vi "configuration UI.vi"() -> ()   [LabVIEW 2013, in "control module editor.lvclass"]
uses:
  control module editor.lvclass
  <vilib>/NI/Configuration Framework/Node/NodeRef.ctl
  <vilib>/NI/Configuration Framework/Node/NISE_CEF_Node.lvclass
  <vilib>/NI/AMC/Message Queue.ctl
  <vilib>/NI/AMC/Message.ctl
  <vilib>/NI/Tools/Keyed Array/KeyedArray.ctl
  <vilib>/NI/Configuration Framework/Node/UserEventRef.ctl
  <vilib>/NI/Configuration Framework/Controls/EventCluster.ctl
  configuration/error classification setting.ctl
  <vilib>/NI/Tag Bus Module Framework/runtime/error classification.ctl
  <vilib>/NI/Configuration Framework/Node/RefreshUIEvent.ctl
  <vilib>/NI/Configuration Framework/Node/CacheState.ctl
  <vilib>/NI/Configuration Framework/Node/StopEvent.ctl
  <vilib>/NI/Configuration Framework/Node/NodeChangeEvent.ctl
  configuration/control module configuration.lvclass
  <vilib>/NI/Configuration Framework/serializable configuration/NISE_CEF_serializable configuration.lvclass/NISE_CEF_serializable configuration.ctl
  <vilib>/NI/Configuration Framework/serializable configuration/NISE_CEF_serializable configuration.lvclass
  configuration/control module configuration.lvclass/control module configuration.ctl
  <vilib>/NI/Tag Bus Module Framework/module configuration/TBM module configuration.lvclass
  <vilib>/NI/Tag Bus Module Framework/channel/TBM channel.lvclass
  <vilib>/NI/Tag Bus/tag/tag descriptor.lvclass/tag descriptor.ctl
  <vilib>/NI/Tag Bus Module Framework/channel/channel classification.ctl
  <vilib>/NI/Configuration Framework/serializable configuration/Read UID.vi
  configuration/Read error classifications.vi
  configuration/Write error classifications.vi
  read fixed channel configuration.vi
  Configuration Editor/Classes/Module editor node/Read Module Configuration.vi
  <vilib>/NI/Module Execution Interface/Engine Configuration/engine configuration.lvclass
  <vilib>/NI/Tag Bus/tag/tag descriptor.lvclass
  <vilib>/NI/Configuration Framework/NISE_CEF_TreeControl.lvlib
  Configuration Editor/Classes/Engine Parent/Engine Parent Editor Node.lvclass
  Configuration Editor/Classes/Module editor node/module editor node.lvclass
  <vilib>/NI/Tools/Keyed Array/Tools_KeyedArray.lvlib
  <vilib>/NI/AMC/AMC.lvlib
  <vilib>/NI/Tag Bus Module Framework/runtime/TBM module execution interface.lvclass
panel:
  in  "node change":T1
  in  "stop event":T2
  in  "cache state":T3
  in  "refresh UI":T4
  in  "Tab Control":T5(tab)
  in  "mapwriters":bool
  out "Channel List":string[][](table)
  in  "mapall":bool
  in  "kvp":i32(listbox)
  in  "error classifications":T6[](array[typedef])
  in  "user event":T8
  in  "main queue":T9
  in  "node ref":T10
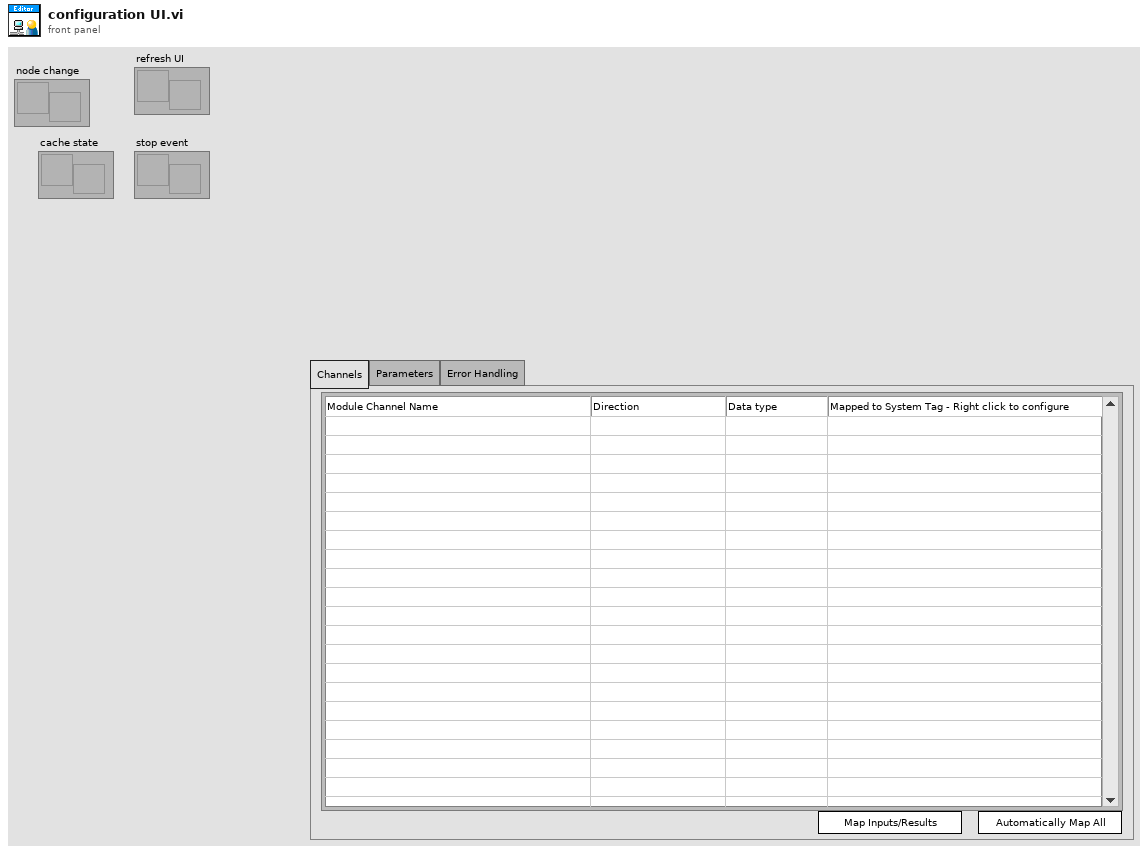
[diagram p1: front panel]
types:
  T1 = typedef "NISE_CEF_Node.lvclass/NodeChangeEvent.ctl" = refnum<user-event>
  T2 = typedef "NISE_CEF_Node.lvclass/StopEvent.ctl" = refnum<user-event>
  T3 = typedef "NISE_CEF_Node.lvclass/CacheState.ctl" = refnum<user-event>
  T4 = typedef "NISE_CEF_Node.lvclass/RefreshUIEvent.ctl" = refnum<user-event>
  T5 = enum32{"Channels", "Parameters", "Error Handling"}
  T6 = typedef "control module configuration.lvclass/error classification setting.ctl" = cluster{"code":i32, "error classification":T7}
  T7 = typedef "TBM module execution interface.lvclass/error classification.ctl" = enum16{"unknown", "none", "trivial", "recoverable", "critical"}
  T8 = typedef "NISE_CEF_Node.lvclass/UserEventRef.ctl" = refnum<user-event>
  T9 = typedef "AMC.lvlib/Message Queue.ctl" = refnum<queue>
  T10 = typedef "NISE_CEF_Node.lvclass/NodeRef.ctl" = refnum<data-value>
  T11 = typedef "control module configuration.lvclass/error classification.ctl" = cluster{"code":i32, "error classification":T7}
  T12 = typedef "NISE_CEF_TreeControl.lvlib/EventCluster.ctl" = cluster{"command":string, "data":string}
  T13 = typedef "LVPoint32TypeDef.ctl" = cluster{"Horizontal":i32, "Vertical":i32}
  T14 = typedef "LVRowAndColumnTypeDef.ctl" = cluster{"Row":i32, "Column":i32}
  T15 = typedef "TBM channel.lvclass/channel classification.ctl" = enum16{"input data", "output data", "processing parameter", "processing result"}
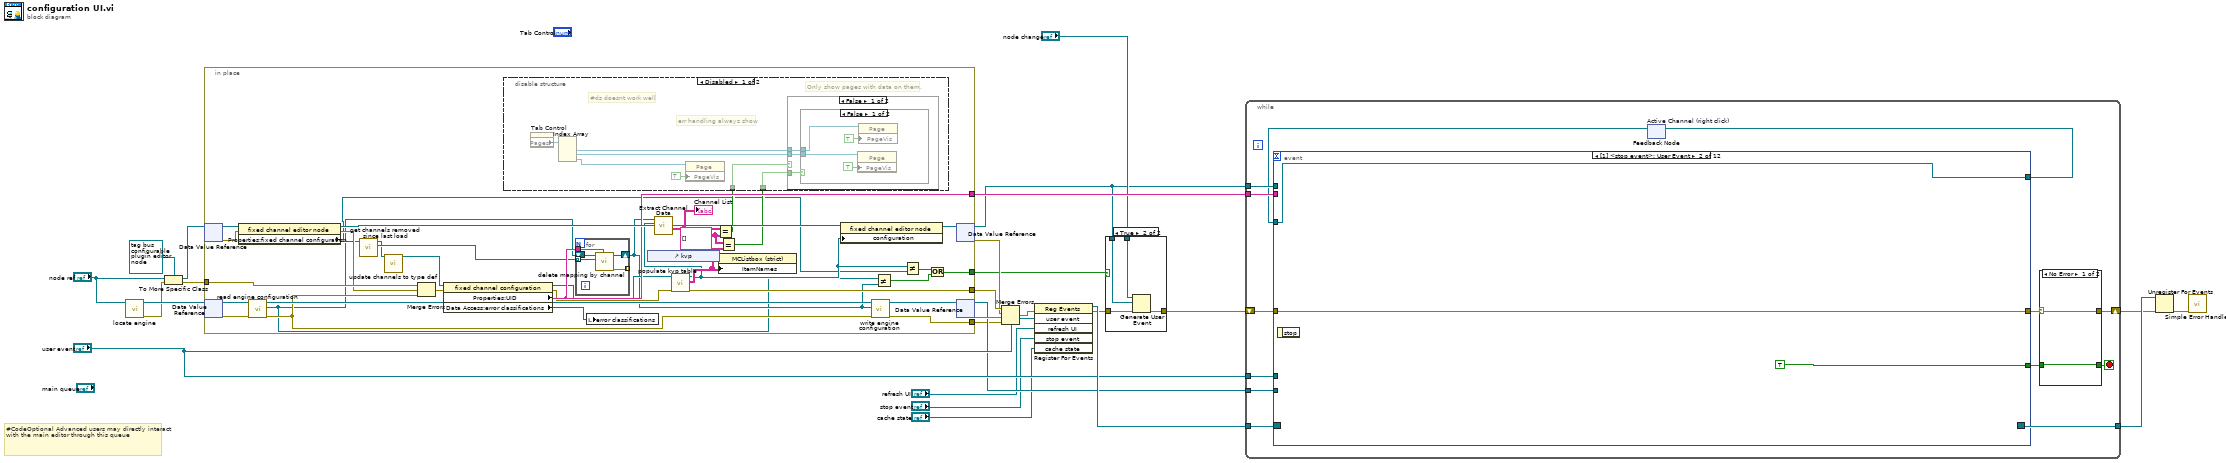
[diagram p0: block diagram]
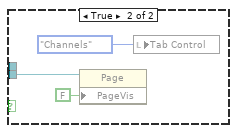
[diagram p3: hidden frame]
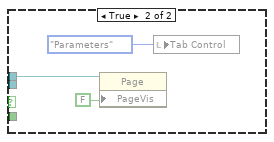
[diagram p4: hidden frame]
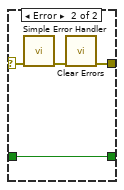
[diagram p6: hidden frame]
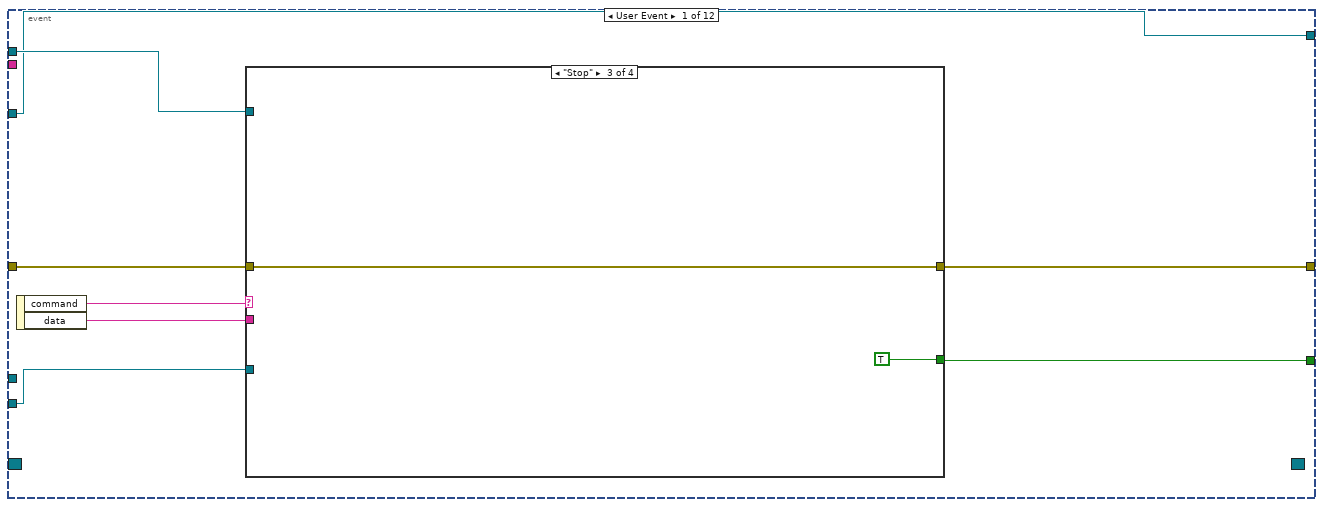
[diagram p7: hidden frame]
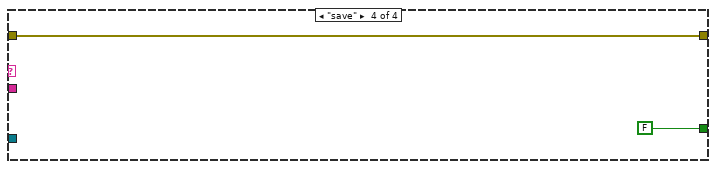
[diagram p10: hidden frame]
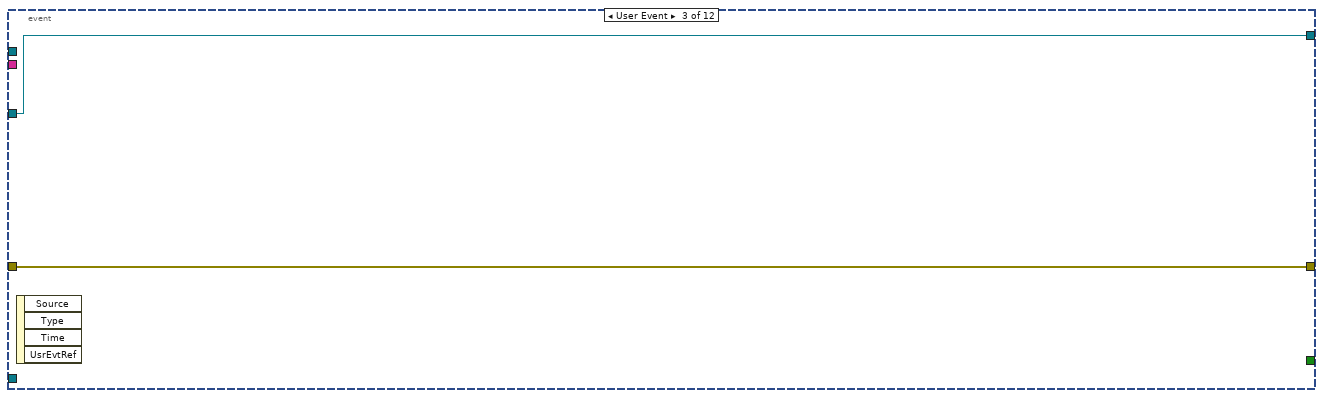
[diagram p11: hidden frame]
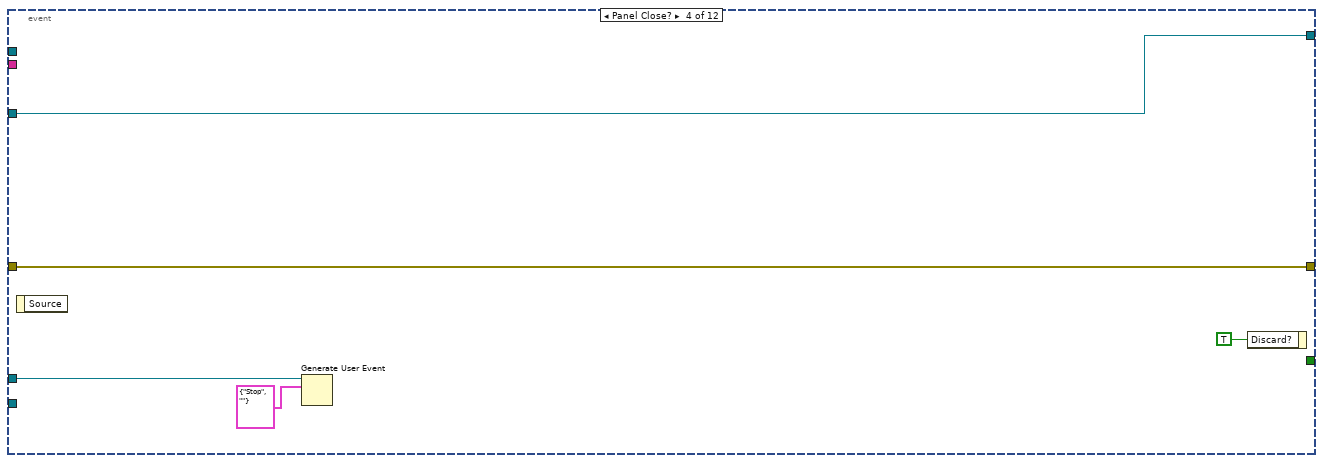
[diagram p12: hidden frame]
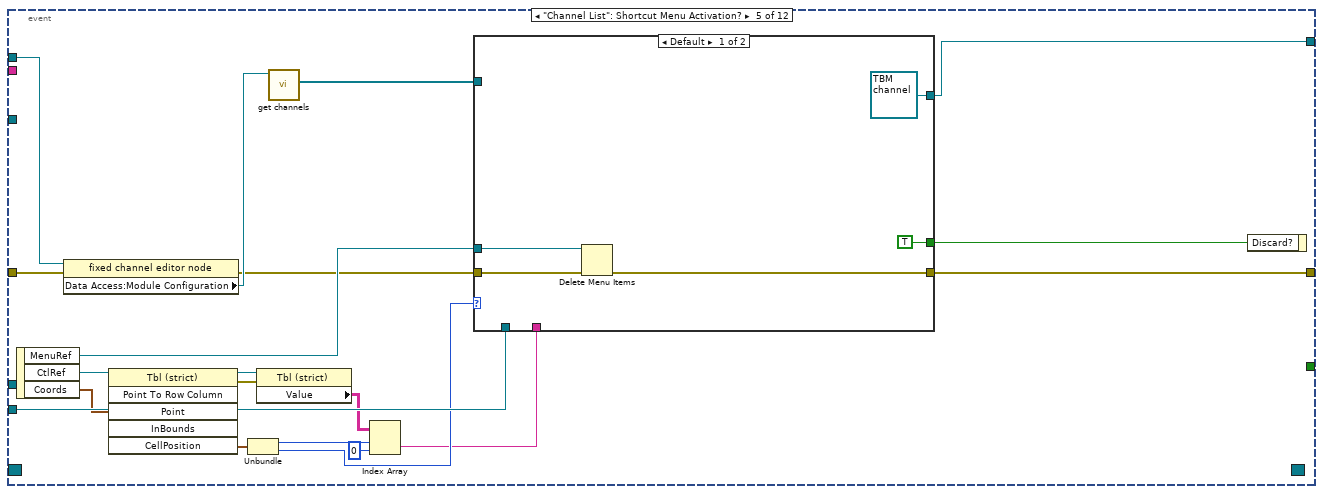
[diagram p13: hidden frame]
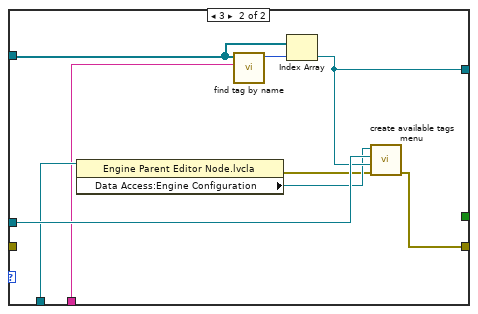
[diagram p14: hidden frame]
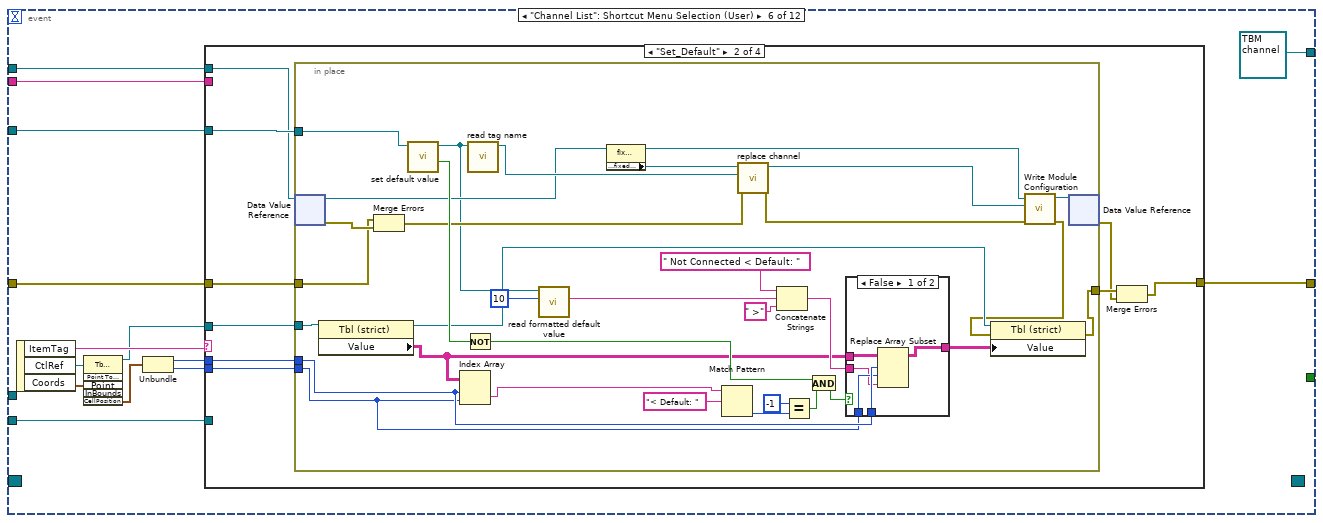
[diagram p15: hidden frame]
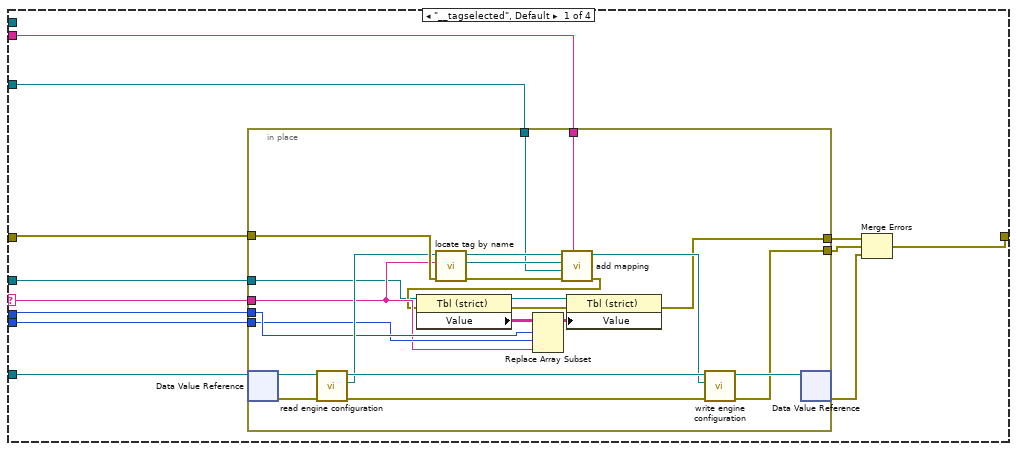
[diagram p16: hidden frame]
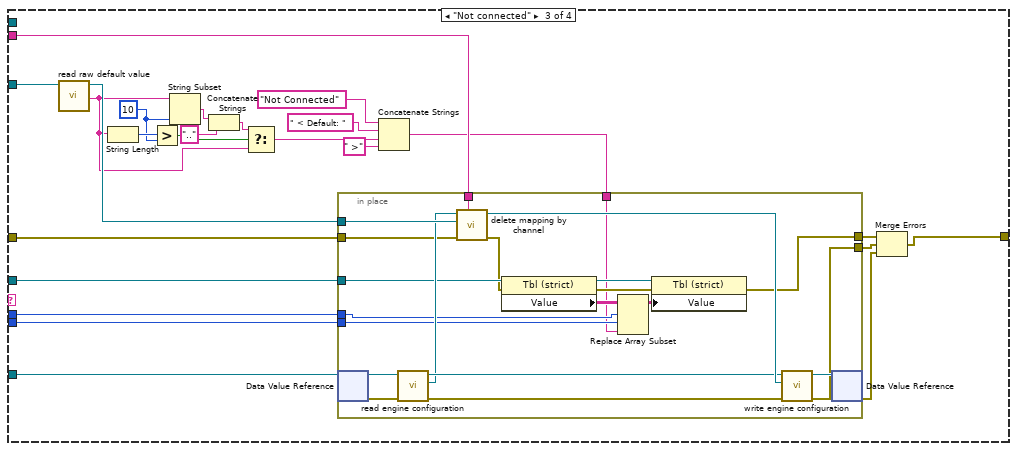
[diagram p18: hidden frame]
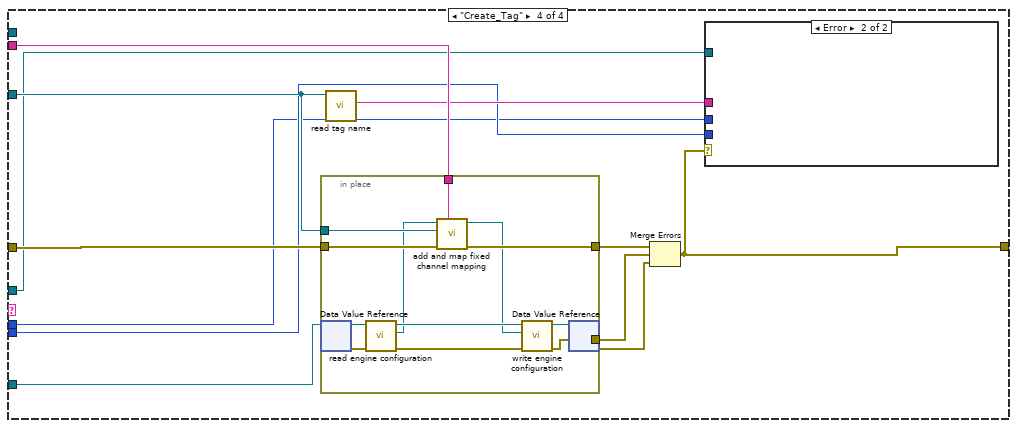
[diagram p19: hidden frame]
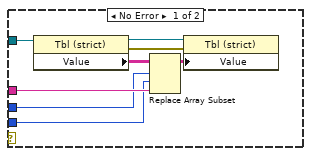
[diagram p20: hidden frame]
diagram:
  # "#CodeOptional Advanced users may directly interact with the main editor through this queue"
  n1 = call "locate engine.vi"("component"="node ref") -> ("error out"=w9:errorcluster, "engine"=w11:refnum<data-value>)  [unwired: 9 in]
  n2 = To More Specific Class(target class=refnum<data-value> refnum ("data value reference"), reference="node ref", error in=w9) -> (specific class reference=w19:refnum<data-value>, error out=w18:errorcluster)
  n3 = in-place {
    in-place-border: w18 -> [w60]
    in-place-border: [w54] -> w17
    in-place-border: [w51] -> w13
    in-place-border: [w35] -> w3
    in-place-border: [w27] -> w2
    w44 = string[][] [] ("y")
    n4 = in-place-dvr #1(w19) -> (w57:refnum<class "control module editor.lvclass">, w52:errorcluster)
    n5 = in-place-dvr #2(w11) -> (w59:refnum<class "Engine Parent Editor Node.lvclass">, w55:errorcluster)
    n6 = property class="fixed channel editor node"(reference=w57, error in=w52) -> (reference out=w53:refnum<class "control module editor.lvclass">, error out=w48:errorcluster, "Properties:fixed channel configuration"=w32:refnum<class "control module configuration.lvclass">)
    n7 = call "read engine configuration.vi"("error in"=w55, "Engine Parent Editor Node in"=w59) -> ("error out"=w36:errorcluster, "engine configuration"=w30:refnum<class "engine configuration.lvclass">, "Engine Parent Editor Node out"=w58:refnum<class "Engine Parent Editor Node.lvclass">)  [unwired: 7 in]
    n8 = call "get channels removed since last load.vi"("fixed channel configuration in"=w32) -> ("removed"=w50:refnum<class "TBM channel.lvclass">[], "fixed channel configuration out"=w40:refnum<class "control module configuration.lvclass">)  [unwired: 9 in]
    n9 = call-dynamic "update channels to type def.vi"("fixed channel configuration in"=w40) -> ("fixed channel configuration out"=w39:refnum<class "control module configuration.lvclass">)  [unwired: 10 in]
    n10 = Merge Errors(w60, w48, w36) -> (w56:errorcluster)
    n11 = property class="fixed channel configuration"(reference=w39, error in=w56) -> (reference out=w34:refnum<class "control module configuration.lvclass">, error out=w49:errorcluster, "Properties:UID"=w51:string, "Data Access:error classifications"=w38:T11[])
    n12 = for {
      tunnel: w51 -> [w85]
      tunnel: w50 -> [w84] mode=indexing
      shift-right: [w83] -> w31
      shift-left: w30 -> [w82]
      tunnel: [w81] -> _ mode=indexing
      n13 = call <vilib>:"delete mapping by channel.vi"("owner ID"=w85, "channel"=w84, "engine configuration in"=w82) -> ("error out"=w81:errorcluster, "engine configuration out"=w83:refnum<class "engine configuration.lvclass">)  [unwired: 7 in]
    }
    n14 = local write "error classifications"(w38) -> ()
    n15 = control-ref of="kvp"() -> (w47:refnum<vi>)
    n16 = call "populate kvp table.vi"("error in"=w49, "fixed channel configuration in"=w34) -> ("error out"=w54:errorcluster, "kvp's"=w43:string[][], "fixed channel configuration out"=w33:refnum<class "control module configuration.lvclass">)  [unwired: 7 in]
    n17 = call "Extract Channel Data.vi"("module configuration in"=w33, "Engine Configuration"=w31) -> ("Channel Data"=w46:string[][])  [unwired: 9 in]
    "Channel List" <- w46
    n18 = Equal?(x=w46, y=w44) -> (x = y?=w45:bool)
    n19 = property on="Property Node" class="MCListbox (strict)"(reference=w47, "ItemNames"=w43) -> ()  [unwired: 1 in, 2 out]
    n20 = Equal?(x=w44, y=w43) -> (x = y?=w42:bool)
    n21 = disable-structure shown="Disabled" {
      disable-tunnel: w45 -> [w66 _]
      disable-tunnel: w42 -> [w64 _]
      frame Disabled {
        # "#ds doesnt work well"
        # "err handling always show"
        # "Only show pages with data on them."
        n22 = property on="Tab Control" class="TabCtl (strict)"() -> ("Pages"=w67:refnum<vi>[])  [unwired: 2 in, 2 out]
        n23 = Index Array(array=w67) -> (element #1=w65:refnum<vi>, element #2=w63:refnum<vi>, element #3=w61:refnum<vi>)  [unwired: 3 in]
        n24 = property class="Page"(reference=w61, "PageVis"=TRUE ("Page Visible")) -> ()  [unwired: 1 in, 2 out]
        n25 = case shown="False" w66 {
          tunnel: w65 -> [w68 w78]
          tunnel: w64 -> [w70 _]
          tunnel: w63 -> [w69 _]
          frame False {
            n26 = case shown="False" w70 {
              tunnel: w69 -> [w71 w75]
              tunnel: w68 -> [w72 _]
              frame False {
                n27 = property class="Page"(reference=w71, "PageVis"=TRUE ("Page Visible")) -> ()  [unwired: 1 in, 2 out]
                n28 = property class="Page"(reference=w72, "PageVis"=TRUE ("Page Visible")) -> ()  [unwired: 1 in, 2 out]
              }
              frame True {
                n29 = property class="Page"(reference=w75, "PageVis"=FALSE ("Page Visible")) -> ()  [unwired: 1 in, 2 out]
                n30 = local write "Tab Control"(enum32{"Channels", "Parameters"}."Channels" ("Tab Control")) -> ()
              }
            }
          }
          frame True {
            n31 = property class="Page"(reference=w78, "PageVis"=FALSE ("Page Visible")) -> ()  [unwired: 1 in, 2 out]
            n32 = local write "Tab Control"(enum32{"Channels", "Parameters"}."Parameters" ("Tab Control")) -> ()
          }
        }
      }
      frame Enabled {
      }
    }
    n33 = property class="fixed channel editor node"(reference=w53, "configuration"=w33) -> (reference out=w41:refnum<class "control module editor.lvclass">)  [unwired: 1 in, 1 out]
    n34 = call "write engine configuration.vi"("error in"=w36, "engine configuration"=w31, "Engine Parent Editor Node in"=w58) -> ("error out"=w35:errorcluster, "Engine Parent Editor Node out"=w37:refnum<class "Engine Parent Editor Node.lvclass">)  [unwired: 7 in]
    n35 = Not Equal?(x=w30, y=w31) -> (x != y?=w28:bool)
    n36 = Not Equal?(x=w33, y=w32) -> (x != y?=w29:bool)
    n37 = Or(x=w29, y=w28) -> (x .or. y?=w27:bool)
    n38 = in-place-dvr #1(w41) -> (w4:refnum<data-value>, w15:errorcluster)
    n39 = in-place-dvr #2(w37) -> (w14:refnum<data-value>, w16:errorcluster)
  }
  n40 = Merge Errors(w17, w15, w16, w3) -> (w12:errorcluster)
  n41 = register-events(error in=w12, "user event", "refresh UI", "stop event", "cache state") -> (reference out=w26:refnum<event-registration>, error out=w22:errorcluster)  [unwired: 1 in]
  n42 = case shown="True" w2 {
    tunnel: w22 -> [w86 w90]
    tunnel: [w86 w89] -> w1
    tunnel: "node change" -> [_ w88]
    tunnel: w4 -> [_ w87]
    frame False {
    }
    frame True {
      n43 = Generate User Event(user event=w88, event data cluster=w87, error in=w90) -> (error out=w89:errorcluster)  [unwired: 1 in, 1 out]
    }
  }
  n44 = while {
    tunnel: w26 -> [w103]
    tunnel: [w102] -> w25
    shift-right: [w98] -> w24
    shift-left: w1 -> [w101]
    tunnel: w13 -> [w97]
    tunnel: w4 -> [w96]
    tunnel: w14 -> [w95]
    tunnel: "user event" -> [w92]
    stop <- w99 stop-if-true
    n45 = feedback #3 "Active Channel (right click)"() -> (w93:refnum<class "TBM channel.lvclass">)  [unwired: 1 in]
    n46 = event shown="[1] <stop event>: User Event" {
      selector: w103 -> [_ _ _ _ _ _ _ _ _ _ _ _]
      dyn-events: [_ _ _ _ _ _ _ _ _ _ _ _] -> w102
      timeout: _ -> [_ _ _ _ _ _ _ _ _ _ _ _]
      tunnel: [w116 TRUE _ _ _ _ _ _ _ _ _ _] -> w91
      tunnel: [w117 w126 w128 w133 w135 w177 w344 w379 w414 w452 w469 w471] -> w100
      tunnel: w101 -> [w111 w126 w128 w133 w153 w178 w348 w382 w418 w453 w469 w471]
      tunnel: w97 -> [_ _ _ _ _ w176 w353 w387 _ _ _ _]
      tunnel: w96 -> [w114 _ _ _ w150 w174 w347 w381 w410 w451 _ _]
      tunnel: w95 -> [w113 _ _ _ w151 w175 w349 w383 _ _ _ _]
      tunnel: w93 -> [w110 w124 w127 w132 _ w179 w354 w388 w420 w454 w468 w470]
      tunnel: [w110 w124 w127 w132 w152 refnum<class "TBM channel.lvclass"> refnum ("channel") w354 w388 w420 w454 w468 w470] -> w94
      tunnel: w92 -> [_ _ _ w130 _ _ _ _ _ _ _ _]
      event User Event {
        n47 = event-data() -> ("command"=w115:string, "data"=w112:string)  [unwired: 1 in]
        n48 = case shown="\"Stop\"" w115 {
          tunnel: [_ _ TRUE FALSE] -> w116
          tunnel: w113 -> [_ _ _ _]
          tunnel: w111 -> [w118 w119 w120 w122]
          tunnel: [w118 w119 w120 w122] -> w117
          tunnel: w114 -> [_ _ _ _]
          tunnel: w112 -> [_ _ _ _]
          frame Default {
          }
          frame "Refresh" {
          }
          frame "Stop" {
          }
          frame "save" {
          }
        }
      }
      event User Event {
        n49 = event-data() -> ()  [unwired: 1 in, 1 out]
      }
      event User Event {
        n50 = event-data() -> ()  [unwired: 1 in, 4 out]
      }
      event Panel Close? {
        n51 = event-data() -> ()  [unwired: 1 in, 1 out]
        n52 = Generate User Event(user event=w130, event data cluster=T12 {"command"="Stop", "data"=""} ("event data")) -> ()  [unwired: 2 in, 2 out]
        n53 = event-data("Discard?"=TRUE) -> ()  [unwired: 1 in, 1 out]
      }
      event "Channel List": Shortcut Menu Activation? {
        n54 = event-data() -> ("MenuRef"=w146:refnum<k9>, "CtlRef"=w147:refnum<vi>, "Coords"=w145:T13)  [unwired: 1 in]
        n55 = property class="fixed channel editor node"(reference=w150, error in=w153) -> (error out=w136:errorcluster, "Data Access:Module Configuration"=w149:refnum<class "TBM module configuration.lvclass">)  [unwired: 1 out]
        n56 = invoke class="Tbl (strict)" method="Point To Row Column"(reference=w147, "Point"=w145) -> (reference out=w143:refnum<vi>, error out=w142:errorcluster, "CellPosition"=w144:T14)  [unwired: 4 in, 3 out]
        n57 = Unbundle(w144) -> ("Row"=w140:i32, "Column"=w138:i32)
        n58 = property class="Tbl (strict)"(reference=w143, error in=w142) -> ("Value"=w141:string[][])  [unwired: 2 out]
        n59 = call-dynamic "get channels.vi"("module configuration in"=w149) -> ("channels"=w148:refnum<class "TBM channel.lvclass">[])  [unwired: 9 in, 1 out]
        n60 = Index Array(array=w141, index (row)=w140, index (col)=0 ("disabled index (col)")) -> (element=w137:string)
        n61 = case shown="Default" w138 {
          tunnel: w146 -> [w157 w167]
          tunnel: [w155 w159] -> w135
          tunnel: w148 -> [_ w161]
          tunnel: [refnum<class "TBM channel.lvclass"> refnum ("channel") w166] -> w152
          tunnel: w151 -> [_ w164]
          tunnel: w137 -> [_ w162]
          tunnel: w136 -> [w156 _]
          tunnel: [TRUE _] -> w134
          frame Default {
            n62 = Delete Menu Items(6:w156, 9:w157) -> (0:w155:errorcluster)  [unwired: 2 in, 1 out]
          }
          frame 3 {
            n63 = property class="Engine Parent Editor Node.lvcla"(reference=w164) -> (error out=w160:errorcluster, "Data Access:Engine Configuration"=w163:refnum<class "engine configuration.lvclass">)  [unwired: 1 in, 1 out]
            n64 = call <vilib>:"find tag by name.vi"("name"=w162, "tags in"=w161) -> ("index"=w165:i32)  [unwired: 9 in]
            n65 = Index Array(array=w161, index=w165) -> (element=w166:refnum<class "TBM channel.lvclass">)
            n66 = call "create available tags menu.vi"("error in"=w160, "channel to map to"=w166, "MenuRef"=w167, "engine configuration in"=w163) -> ("error out"=w159:errorcluster)  [unwired: 6 in, 1 out]
          }
        }
        n67 = event-data("Discard?"=w134) -> ()  [unwired: 1 in, 1 out]
      }
      event "Channel List": Shortcut Menu Selection (User) {
        n68 = event-data() -> ("ItemTag"=w181:string, "CtlRef"=w173:refnum<vi>, "Coords"=w172:T13)  [unwired: 1 in]
        n69 = invoke class="Tbl (strict)" method="Point To Row Column"(reference=w173, "Point"=w172) -> (reference out=w168:refnum<vi>, "CellPosition"=w171:T14)  [unwired: 4 in, 4 out]
        n70 = Unbundle(w171) -> ("Row"=w170:i32, "Column"=w169:i32)
        n71 = case shown="\"Set_Default\"" w181 {
          selector: w181 -> [w191 _ _ _]
          tunnel: w169 -> [w193 w225 w289 w313]
          tunnel: w170 -> [w192 w224 w288 w312]
          tunnel: w179 -> [w189 w226 w284 w316]
          tunnel: [w186 w222 w269 w314] -> w177
          tunnel: w178 -> [w190 w218 w287 w322]
          tunnel: w176 -> [w187 _ w285 w320]
          tunnel: w175 -> [w183 _ w270 w319]
          tunnel: w174 -> [_ w223 _ _]
          tunnel: w168 -> [w182 w219 w266 w311]
          frame "__tagselected", Default {
            n72 = in-place {
              in-place-border: w193 -> [w198]
              in-place-border: w192 -> [w199]
              in-place-border: w191 -> [w197]
              in-place-border: w190 -> [w217]
              in-place-border: w189 -> [w214]
              in-place-border: [w195] -> w188
              in-place-border: w187 -> [w212]
              in-place-border: [w206] -> w184
              in-place-border: w182 -> [w194]
              n73 = in-place-dvr #4(w183) -> (w209:refnum<class "Engine Parent Editor Node.lvclass">, w208:errorcluster)
              n74 = call "read engine configuration.vi"("error in"=w208, "Engine Parent Editor Node in"=w209) -> ("error out"=w210:errorcluster, "engine configuration"=w204:refnum<class "engine configuration.lvclass">, "Engine Parent Editor Node out"=w211:refnum<class "Engine Parent Editor Node.lvclass">)  [unwired: 7 in]
              n75 = call <vilib>:"locate tag by name.vi"("error in"=w217, "tag name"=w197, "engine configuration in"=w204) -> ("error out"=w213:errorcluster, "tag descriptor"=w215:refnum<class "tag descriptor.lvclass">, "engine configuration out"=w216:refnum<class "engine configuration.lvclass">)  [unwired: 6 in]
              n76 = call <vilib>:"add mapping.vi"("owner ID"=w212, "error in"=w213, "channel"=w214, "tag descriptor"=w215, "engine configuration"=w216) -> ("error out"=w196:errorcluster, "engine configuration out"=w205:refnum<class "engine configuration.lvclass">)  [unwired: 5 in]
              n77 = property class="Tbl (strict)"(reference=w194, error in=w196) -> (reference out=w201:refnum<vi>, error out=w202:errorcluster, "Value"=w200:string[][])
              n78 = Replace Array Subset(array=w200, new element=w197, index (row)=w199, index (col)=w198) -> (w203:string[][])
              n79 = property class="Tbl (strict)"(reference=w201, error in=w202, "Value"=w203) -> (error out=w195:errorcluster)  [unwired: 1 out]
              n80 = call "write engine configuration.vi"("error in"=w210, "engine configuration"=w205, "Engine Parent Editor Node in"=w211) -> ("error out"=w206:errorcluster, "Engine Parent Editor Node out"=w207:refnum<class "Engine Parent Editor Node.lvclass">)  [unwired: 7 in]
              n81 = in-place-dvr #4(w207) -> (w185:errorcluster)  [unwired: 1 out]
            }
            n82 = Merge Errors(w188, w184, w185) -> (w186:errorcluster)
          }
          frame "Set_Default" {
            n83 = in-place {
              in-place-border: w226 -> [w259]
              in-place-border: w225 -> [w237]
              in-place-border: w224 -> [w238]
              in-place-border: [w235] -> w221
              in-place-border: w219 -> [w243]
              in-place-border: w218 -> [w230]
              n84 = in-place-dvr #5(w223) -> (w233:refnum<class "control module editor.lvclass">, w246:errorcluster)
              n85 = property class="Tbl (strict)"(reference=w243) -> (reference out=w241:refnum<vi>, "Value"=w240:string[][])  [unwired: 1 in, 1 out]
              n86 = Merge Errors(w230, w246) -> (w231:errorcluster)
              n87 = call "set default value.vi"("tag"=w259) -> ("cancelled?"=w251:bool, "tag out"=w229:refnum<class "TBM channel.lvclass">)  [unwired: 9 in]
              n88 = Index Array(array=w240, index (row)=w238, index (col)=w237) -> (element=w239:string)
              n89 = Not(x=w251) -> (.not. x?=w249:bool)
              n90 = call <vilib>:"read tag name.vi"("system tag in"=w229) -> ("system tag out"=w244:refnum<class "TBM channel.lvclass">)  [unwired: 8 in, 2 out]
              n91 = call "read formatted default value.vi"("# of Digits"=u8 10, "channel"=w229) -> ("Formatted Default"=w227:string)  [unwired: 8 in, 1 out]
              n92 = property class="fixed channel editor node"(reference=w233) -> (reference out=w232:refnum<class "control module editor.lvclass">, "Properties:fixed channel configuration"=w234:refnum<class "control module configuration.lvclass">)  [unwired: 1 in, 1 out]
              n93 = Match Pattern(string=w239, regular expression="< Default: ") -> (offset past match=w257:i32)  [unwired: 1 in, 3 out]
              n94 = call "replace channel.vi"("error in"=w231, "channel"=w244, "fixed module parent implementation configuration in"=w234) -> ("error out"=w245:errorcluster, "fixed module parent implementation configuration out"=w247:refnum<class "control module configuration.lvclass">)  [unwired: 7 in]
              n95 = Concatenate Strings(" Not Connected < Default: " ("string"), w227, " >" ("string")) -> (w250:string)
              n96 = Equal?(x=-1, y=w257) -> (x = y?=w255:bool)
              n97 = And(x=w249, y=w255) -> (x .and. y?=w252:bool)
              n98 = case shown="False" w252 {
                tunnel: w250 -> [w260 _]
                tunnel: w240 -> [w264 w265]
                tunnel: [w263 w265] -> w242
                tunnel: w238 -> [w262 _]
                tunnel: w237 -> [w261 _]
                frame False {
                  n99 = Replace Array Subset(array=w264, new element=w260, index (row)=w262, index (col)=w261) -> (w263:string[][])
                }
                frame True {
                }
              }
              n100 = call "Write Module Configuration.vi"("error in"=w245, "module configuration"=w247, "Module Editor Node in"=w232) -> ("error out"=w236:errorcluster, "Module Editor Node out"=w248:refnum<class "control module editor.lvclass">)  [unwired: 7 in]
              n101 = property class="Tbl (strict)"(reference=w241, error in=w236, "Value"=w242) -> (error out=w235:errorcluster)  [unwired: 1 out]
              n102 = in-place-dvr #5(w248) -> (w220:errorcluster)  [unwired: 1 out]
            }
            n103 = Merge Errors(w221, w220) -> (w222:errorcluster)
          }
          frame "Not connected" {
            w277 = 10 ("y")
            n104 = call <vilib>:"read raw default value.vi"("system tag in"=w284) -> ("raw default"=w273:string, "system tag out"=w283:refnum<class "TBM channel.lvclass">)  [unwired: 8 in, 1 out]
            n105 = String Length(string=w273) -> (length=w279:i32)
            n106 = Greater?(x=w279, y=w277) -> (0:w278:bool)
            n107 = String Subset(string=w273, length (rest)=w277) -> (substring=w275:string)  [unwired: 1 in]
            n108 = Concatenate Strings(w275, ".." ("string")) -> (w276:string)
            n109 = Select(t=w276, s=w278, f=w273) -> (s? t:f=w272:string)
            n110 = Concatenate Strings("Not Connected" ("string"), " < Default: " ("string"), w272, " >" ("string")) -> (w282:string)
            n111 = in-place {
              in-place-border: w289 -> [w295]
              in-place-border: w288 -> [w296]
              in-place-border: w287 -> [w292]
              in-place-border: [w290] -> w286
              in-place-border: w285 -> [w310]
              in-place-border: w283 -> [w309]
              in-place-border: w282 -> [w293]
              in-place-border: [w304] -> w267
              in-place-border: w266 -> [w294]
              n112 = in-place-dvr #6(w270) -> (w308:refnum<class "Engine Parent Editor Node.lvclass">, w307:errorcluster)
              n113 = call "read engine configuration.vi"("error in"=w307, "Engine Parent Editor Node in"=w308) -> ("error out"=w305:errorcluster, "engine configuration"=w301:refnum<class "engine configuration.lvclass">, "Engine Parent Editor Node out"=w302:refnum<class "Engine Parent Editor Node.lvclass">)  [unwired: 7 in]
              n114 = call <vilib>:"delete mapping by channel.vi"("owner ID"=w310, "error in"=w292, "channel"=w309, "engine configuration in"=w301) -> ("error out"=w291:errorcluster, "engine configuration out"=w303:refnum<class "engine configuration.lvclass">)  [unwired: 6 in]
              n115 = property class="Tbl (strict)"(reference=w294, error in=w291) -> (reference out=w298:refnum<vi>, error out=w299:errorcluster, "Value"=w297:string[][])
              n116 = Replace Array Subset(array=w297, new element=w293, index (row)=w296, index (col)=w295) -> (w300:string[][])
              n117 = property class="Tbl (strict)"(reference=w298, error in=w299, "Value"=w300) -> (error out=w290:errorcluster)  [unwired: 1 out]
              n118 = call "write engine configuration.vi"("error in"=w305, "engine configuration"=w303, "Engine Parent Editor Node in"=w302) -> ("error out"=w304:errorcluster, "Engine Parent Editor Node out"=w306:refnum<class "Engine Parent Editor Node.lvclass">)  [unwired: 7 in]
              n119 = in-place-dvr #6(w306) -> (w268:errorcluster)  [unwired: 1 out]
            }
            n120 = Merge Errors(w286, w267, w268) -> (w269:errorcluster)
          }
          frame "Create_Tag" {
            n121 = in-place {
              in-place-border: w322 -> [w342]
              in-place-border: [w341] -> w321
              in-place-border: w320 -> [w340]
              in-place-border: w316 -> [w339]
              in-place-border: [w335] -> w317
              n122 = in-place-dvr #7(w319) -> (w337:refnum<class "Engine Parent Editor Node.lvclass">, w338:errorcluster)
              n123 = call "read engine configuration.vi"("error in"=w338, "Engine Parent Editor Node in"=w337) -> ("error out"=w334:errorcluster, "engine configuration"=w332:refnum<class "engine configuration.lvclass">, "Engine Parent Editor Node out"=w333:refnum<class "Engine Parent Editor Node.lvclass">)  [unwired: 7 in]
              n124 = call <vilib>:"add and map fixed channel mapping.vi"("module instance"=w340, "error in"=w342, "fixed channel"=w339, "engine configuration in"=w332) -> ("error out"=w341:errorcluster, "engine configuration out"=w331:refnum<class "engine configuration.lvclass">)  [unwired: 6 in]
              n125 = call "write engine configuration.vi"("error in"=w334, "engine configuration"=w331, "Engine Parent Editor Node in"=w333) -> ("error out"=w335:errorcluster, "Engine Parent Editor Node out"=w336:refnum<class "Engine Parent Editor Node.lvclass">)  [unwired: 7 in]
              n126 = in-place-dvr #7(w336) -> (w318:errorcluster)  [unwired: 1 out]
            }
            n127 = call <vilib>:"read tag name.vi"("system tag in"=w316) -> ("name"=w315:string)  [unwired: 8 in, 2 out]
            n128 = Merge Errors(w321, w317, w318) -> (w314:errorcluster)
            n129 = case shown="Error" w314 {
              tunnel: w315 -> [w326 _]
              tunnel: w313 -> [w325 _]
              tunnel: w312 -> [w324 _]
              tunnel: w311 -> [w323 _]
              frame No Error {
                n130 = property class="Tbl (strict)"(reference=w323) -> (reference out=w328:refnum<vi>, error out=w329:errorcluster, "Value"=w327:string[][])  [unwired: 1 in]
                n131 = Replace Array Subset(array=w327, new element=w326, index (row)=w324, index (col)=w325) -> (w330:string[][])
                n132 = property class="Tbl (strict)"(reference=w328, error in=w329, "Value"=w330) -> ()  [unwired: 2 out]
              }
              frame Error {
              }
            }
          }
        }
      }
      event "mapall": Value Change {
        n133 = event-data() -> ()  [unwired: 1 in, 1 out]
        n134 = property class="fixed channel editor node"(reference=w347) -> ("Data Access:Module Configuration"=w346:refnum<class "TBM module configuration.lvclass">)  [unwired: 1 in, 2 out]
        n135 = call-dynamic "get channels.vi"("module configuration in"=w346) -> ("channels"=w345:refnum<class "TBM channel.lvclass">[], "module configuration out"=w343:refnum<class "TBM module configuration.lvclass">)  [unwired: 9 in]
        n136 = in-place {
          in-place-border: [w368] -> w352
          in-place-border: [w364] -> w351
          in-place-border: w353 -> [w360]
          in-place-border: w348 -> [w359]
          in-place-border: w345 -> [w358]
          in-place-border: w343 -> [w355]
          n137 = in-place-dvr #8(w349) -> (w366:refnum<class "Engine Parent Editor Node.lvclass">, w367:errorcluster)
          n138 = call "read engine configuration.vi"("error in"=w367, "Engine Parent Editor Node in"=w366) -> ("error out"=w363:errorcluster, "engine configuration"=w361:refnum<class "engine configuration.lvclass">, "Engine Parent Editor Node out"=w362:refnum<class "Engine Parent Editor Node.lvclass">)  [unwired: 7 in]
          n139 = for {
            tunnel: [w374] -> w368 mode=indexing
            tunnel: w360 -> [w371]
            tunnel: w359 -> [w370]
            shift-right: [w372] -> w356
            shift-left: w361 -> [w373]
            tunnel: w358 -> [w369] mode=indexing
            n140 = call <vilib>:"add and map fixed channel mapping.vi"("module instance"=w371, "error in"=w370, "fixed channel"=w369, "engine configuration in"=w373) -> ("error out"=w374:errorcluster, "engine configuration out"=w372:refnum<class "engine configuration.lvclass">)  [unwired: 6 in]
          }
          n141 = call "write engine configuration.vi"("error in"=w363, "engine configuration"=w356, "Engine Parent Editor Node in"=w362) -> ("error out"=w364:errorcluster, "Engine Parent Editor Node out"=w365:refnum<class "Engine Parent Editor Node.lvclass">)  [unwired: 7 in]
          n142 = call "Extract Channel Data.vi"("module configuration in"=w355, "Engine Configuration"=w356) -> ("Channel Data"=w357:string[][])  [unwired: 9 in]
          n143 = local write "Channel List"(w357) -> ()
          n144 = in-place-dvr #8(w365) -> (w350:errorcluster)  [unwired: 1 out]
        }
        n145 = Merge Errors(w352, w351, w350) -> (w344:errorcluster)
      }
      event "mapwriters": Value Change {
        w377 = T15[] [enum."input data", enum."processing result"] items=["input data", "output data", "processing parameter", "processing result"] ("allowed classifications")
        n146 = event-data() -> ()  [unwired: 1 in, 1 out]
        n147 = property class="fixed channel editor node"(reference=w381) -> ("Data Access:Module Configuration"=w380:refnum<class "TBM module configuration.lvclass">)  [unwired: 1 in, 2 out]
        n148 = call-dynamic "get channels.vi"("module configuration in"=w380) -> ("channels"=w376:refnum<class "TBM channel.lvclass">[], "module configuration out"=w378:refnum<class "TBM module configuration.lvclass">)  [unwired: 9 in]
        n149 = call <vilib>:"filter channels by classification.vi"("allowed classifications"=w377, "channels in"=w376) -> ("channels out"=w375:refnum<class "TBM channel.lvclass">[])  [unwired: 9 in]
        n150 = in-place {
          in-place-border: [w402] -> w386
          in-place-border: [w398] -> w385
          in-place-border: w387 -> [w394]
          in-place-border: w382 -> [w393]
          in-place-border: w375 -> [w392]
          in-place-border: w378 -> [w389]
          n151 = in-place-dvr #9(w383) -> (w400:refnum<class "Engine Parent Editor Node.lvclass">, w401:errorcluster)
          n152 = call "read engine configuration.vi"("error in"=w401, "Engine Parent Editor Node in"=w400) -> ("error out"=w397:errorcluster, "engine configuration"=w395:refnum<class "engine configuration.lvclass">, "Engine Parent Editor Node out"=w396:refnum<class "Engine Parent Editor Node.lvclass">)  [unwired: 7 in]
          n153 = for {
            tunnel: [w408] -> w402 mode=indexing
            tunnel: w394 -> [w405]
            tunnel: w393 -> [w404]
            shift-right: [w406] -> w390
            shift-left: w395 -> [w407]
            tunnel: w392 -> [w403] mode=indexing
            n154 = call <vilib>:"add and map fixed channel mapping.vi"("module instance"=w405, "error in"=w404, "fixed channel"=w403, "engine configuration in"=w407) -> ("error out"=w408:errorcluster, "engine configuration out"=w406:refnum<class "engine configuration.lvclass">)  [unwired: 6 in]
          }
          n155 = call "write engine configuration.vi"("error in"=w397, "engine configuration"=w390, "Engine Parent Editor Node in"=w396) -> ("error out"=w398:errorcluster, "Engine Parent Editor Node out"=w399:refnum<class "Engine Parent Editor Node.lvclass">)  [unwired: 7 in]
          n156 = call "Extract Channel Data.vi"("module configuration in"=w389, "Engine Configuration"=w390) -> ("Channel Data"=w391:string[][])  [unwired: 9 in]
          n157 = local write "Channel List"(w391) -> ()
          n158 = in-place-dvr #9(w399) -> (w384:errorcluster)  [unwired: 1 out]
        }
        n159 = Merge Errors(w386, w385, w384) -> (w379:errorcluster)
      }
      event "kvp": Edit Cell? {
        n160 = event-data() -> ("CtlRef"=w419:refnum<vi>, "Coords"=w409:T14, "String"=w411:string)  [unwired: 1 in]
        n161 = property class="MCListbox (strict)"(reference=w419, error in=w418) -> (error out=w415:errorcluster, "ItemNames"=w413:string[][])  [unwired: 1 out]
        n162 = Unbundle By Name(w409) -> ("Row"=w412:i32, "Column"=w417:i32)
        n163 = case shown="1, Default" w417 {
          tunnel: [w425 TRUE] -> w416
          tunnel: w415 -> [w428 w446]
          tunnel: [w426 w446] -> w414
          tunnel: w413 -> [w424 _]
          tunnel: w412 -> [w423 _]
          tunnel: w411 -> [w422 _]
          tunnel: w410 -> [w429 _]
          frame 1, Default {
            n164 = in-place {
              in-place-border: w428 -> [w445]
              in-place-border: w424 -> [w444]
              in-place-border: w423 -> [w442]
              in-place-border: w422 -> [w440]
              in-place-border: [w430] -> w421
              n165 = in-place-dvr #10(w429) -> (w438:refnum<class "control module editor.lvclass">, w436:errorcluster)
              n166 = Index Array(array=w444, index (row)=w442, index (col)=0 ("disabled index (col)")) -> (element=w441:string)
              n167 = property class="fixed channel editor node"(reference=w438, error in=w436) -> (reference out=w433:refnum<class "control module editor.lvclass">, error out=w435:errorcluster, "Properties:fixed channel configuration"=w437:refnum<class "control module configuration.lvclass">)
              n168 = Merge Errors(w445, w435) -> (w439:errorcluster)
              n169 = call-dynamic "set value for key.vi"("error in"=w439, "value"=w440, "key"=w441, "fixed channel configuration in"=w437) -> ("error out"=w434:errorcluster, "fixed channel configuration out"=w431:refnum<class "control module configuration.lvclass">)  [unwired: 6 in]
              n170 = property class="fixed channel editor node"(reference=w433, error in=w434, "configuration"=w431) -> (reference out=w432:refnum<class "control module editor.lvclass">, error out=w430:errorcluster)
              n171 = in-place-dvr #10(w432) -> (w427:errorcluster)  [unwired: 1 out]
            }
            n172 = Merge Errors(w421, w427) -> (w426:errorcluster)
            n173 = Unbundle By Name(w426) -> ("status"=w425:bool)
          }
          frame ..0 {
          }
        }
        n174 = event-data("Discard?"=w416) -> ()  [unwired: 1 in, 1 out]
      }
      event "error classifications": Value Change {
        n175 = event-data() -> ()  [unwired: 1 in, 3 out]
        n176 = in-place {
          in-place-border: w453 -> [w466]
          in-place-border: [w460] -> w449
          in-place-border: "error classifications" -> [w455]
          n177 = in-place-dvr #11(w451) -> (w465:refnum<class "control module editor.lvclass">, w464:errorcluster)
          n178 = property class="fixed channel editor node"(reference=w465, error in=w464) -> (reference out=w462:refnum<class "control module editor.lvclass">, error out=w463:errorcluster, "Properties:fixed channel configuration"=w459:refnum<class "control module configuration.lvclass">)
          n179 = Merge Errors(w466, w463) -> (w458:errorcluster)
          n180 = property class="fixed channel configuration"(reference=w459, error in=w458, "Data Access:error classifications"=w455) -> (reference out=w456:refnum<class "control module configuration.lvclass">, error out=w457:errorcluster)
          n181 = property class="fixed channel editor node"(reference=w462, error in=w457, "configuration"=w456) -> (reference out=w461:refnum<class "control module editor.lvclass">, error out=w460:errorcluster)
          n182 = in-place-dvr #11(w461) -> (w450:errorcluster)  [unwired: 1 out]
        }
        n183 = Merge Errors(w449, w450) -> (w452:errorcluster)
      }
      event "kvp": Shortcut Menu Activation? {
        # "Igore the right-click menu"
        n184 = event-data() -> ()  [unwired: 1 in, 1 out]
        n185 = event-data("Discard?"=TRUE) -> ()  [unwired: 1 in, 1 out]
      }
      event Pane Size {
        n186 = event-data() -> ()  [unwired: 1 in, 1 out]
      }
    }
    n187 = feedback-in #3(w94) -> ()
    n188 = case shown="No Error" w100 {
      selector: w100 -> [w104 w107]
      tunnel: [w105 w109] -> w99
      tunnel: w91 -> [w105 w109]
      tunnel: [w104 w108] -> w98
      frame No Error {
      }
      frame Error {
        n189 = call <vilib>:"Simple Error Handler.vi"("error in (no error)"=w107) -> ("error out"=w106:errorcluster)  [unwired: 4 in, 4 out]
        n190 = call <vilib>:"Clear Errors.vi"("error in (no error)"=w106) -> ("error out"=w108:errorcluster)  [unwired: 6 in]
      }
    }
  }
  n191 = Unregister For Events(event registration refnum=w25, error in=w24) -> (error out=w21:errorcluster)
  n192 = call <vilib>:"Simple Error Handler.vi"("error in (no error)"=w21) -> ()  [unwired: 4 in, 5 out]
